vi "objectDB.vi"(7 "Action":T1, 8 "error in (no error)":errorcluster, 9 "timeout in ms (0)":i32, 10 "name":string, 11 "objectRef":refnum<class "HGF_Reference.lvclass">) -> (0 "error out":errorcluster, 1 "obj exists":bool, 2 "name out":string, 3 "objectRef out":refnum<class "HGF_Reference.lvclass">, 4 "object list names":string[](array[string]), 5 "object list refs":refnum<class "HGF_Reference.lvclass">[](array[class]))   [LabVIEW 2012, in "HGF_ObjectManager.lvlib"]
doc: "Functional Global Variable that manages an array of referenced objects by name."
uses:
  HGF_ObjectManager.lvlib
  HGF_BaseClasses/HGF_Reference/HGF_Reference.lvclass
  action.ctl
panel:
  in  "objectType":T2
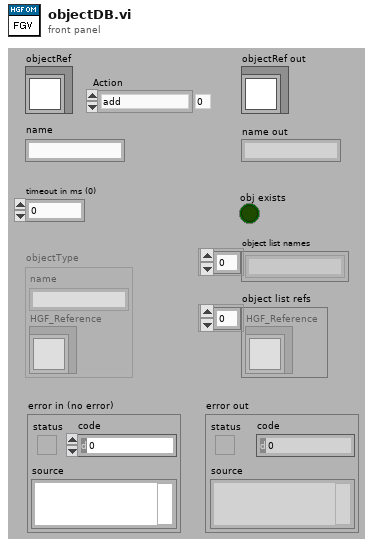
[diagram p1: front panel]
types:
  T1 = typedef "HGF_ObjectManager.lvlib/action.ctl" = enum16{"add", "remove", "name2ref", "ref2name ", "obj exists?", "cleanup", "get object list", "reset"}
  T2 = cluster{"name":string, "HGF_Reference":refnum<class "HGF_Reference.lvclass">}
  T3 = cluster{"name":string, "HGF_Reference":refnum<class "HGF_Reference.lvclass">}[]
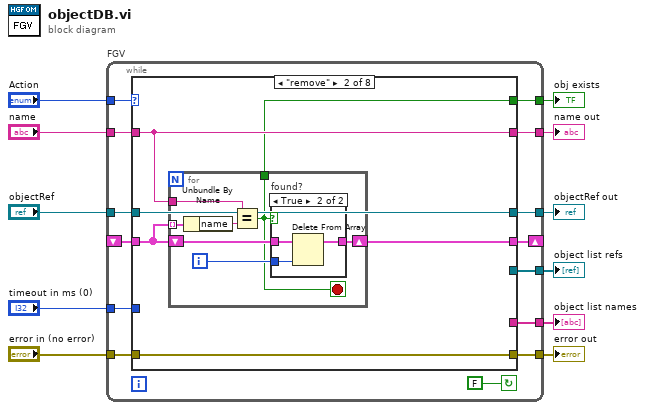
[diagram p0: block diagram]
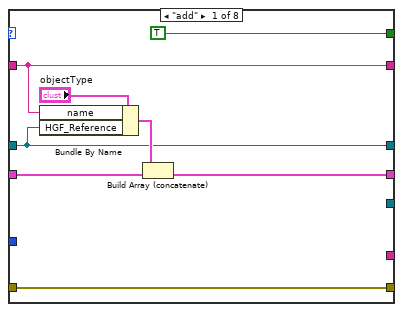
[diagram p2: hidden frame]
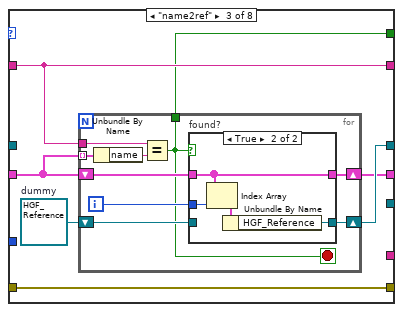
[diagram p4: hidden frame]
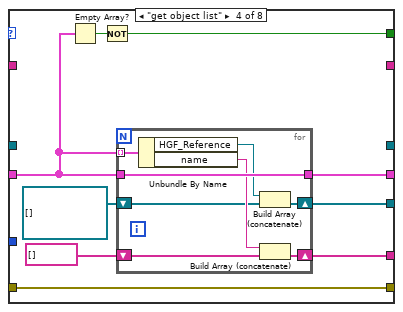
[diagram p6: hidden frame]
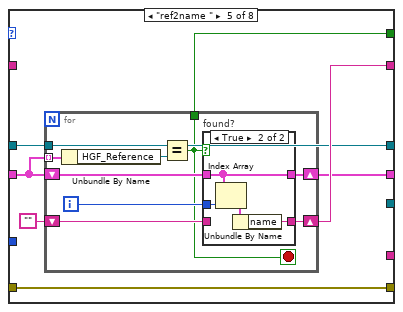
[diagram p7: hidden frame]
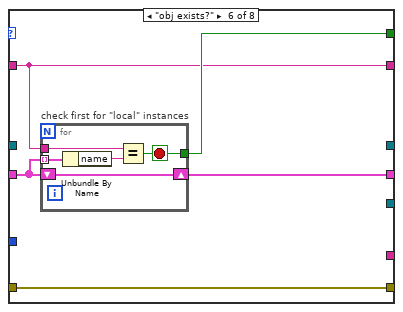
[diagram p9: hidden frame]
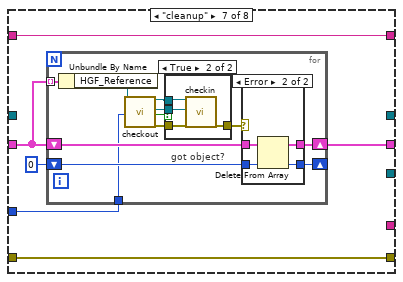
[diagram p10: hidden frame]
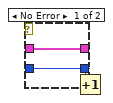
[diagram p12: hidden frame]
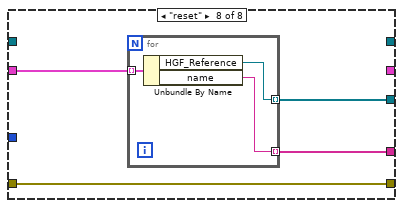
[diagram p13: hidden frame]
diagram:
  n1 = while "FGV" {
    shift-right: [w15] -> _
    shift-left: _ -> [w23]
    tunnel: "name" -> [w25]
    tunnel: "objectRef" -> [w24]
    tunnel: "Action" -> [w22]
    tunnel: [w21] -> w8
    tunnel: [w20] -> w9
    tunnel: [w18] -> w4
    tunnel: [w17] -> w10
    tunnel: [w16] -> w11
    tunnel: "timeout in ms (0)" -> [w14]
    tunnel: "error in (no error)" -> [w13]
    tunnel: [w12] -> w1
    stop <- FALSE continue-if-true
    n2 = case shown="\"remove\"" w22 {
      tunnel: w25 -> [w29 w37 w54 _ _ w113 w124 _]
      tunnel: w24 -> [w30 w36 _ _ w91 _ _ _]
      tunnel: w23 -> [w32 w39 w56 w75 w93 w116 w127 w154]
      tunnel: [w30 w36 w57 _ w91 _ _ _] -> w21
      tunnel: [w29 w37 w54 _ w95 w113 w124 _] -> w20
      tunnel: [TRUE w35 w52 w73 w92 w114 _ _] -> w18
      tunnel: [_ _ _ w79 _ _ _ w152] -> w17
      tunnel: [_ _ _ w78 _ _ _ w153] -> w16
      tunnel: [w31 w38 w55 w81 w94 w115 w126 _] -> w15
      tunnel: w14 -> [_ _ _ _ _ _ w123 _]
      tunnel: w13 -> [w26 w34 w51 w76 w90 w112 w122 w151]
      tunnel: [w26 w34 w51 w76 w90 w112 w122 w151] -> w12
      frame "add" {
        n3 = Bundle By Name(cluster="objectType", "name"=w29, "HGF_Reference"=w30) -> (w33:T2)
        n4 = Build Array (concatenate)(w33, w32) -> (w31:T3)
      }
      frame "remove" {
        n5 = for {
          tunnel: w39 -> [w46] mode=indexing
          tunnel: w37 -> [w45]
          shift-right: [w41] -> w38
          shift-left: w39 -> [w42]
          tunnel: [w40] -> w35
          i -> [w43]
          stop <- w40 stop-if-true
          n6 = Unbundle By Name(w46) -> ("name"=w44:string)
          n7 = Equal?(x=w45, y=w44) -> (x = y?=w40:bool)
          n8 = case "found?" shown="True" w40 {
            tunnel: w42 -> [w47 w50]
            tunnel: w43 -> [_ w48]
            tunnel: [w47 w49] -> w41
            frame False {
            }
            frame True {
              n9 = Delete From Array(array=w50, index=w48) -> (array with subset deleted=w49:T3)  [unwired: 1 in, 1 out]
            }
          }
        }
      }
      frame "name2ref" {
        w53 = refnum<class "HGF_Reference.lvclass"> refnum  # dummy
        n10 = for {
          tunnel: w56 -> [w66] mode=indexing
          tunnel: w54 -> [w65]
          shift-right: [w62] -> w57
          shift-left: w53 -> [w61]
          shift-right: [w60] -> w55
          shift-left: w56 -> [w59]
          tunnel: [w58] -> w52
          i -> [w63]
          stop <- w58 stop-if-true
          n11 = Unbundle By Name(w66) -> ("name"=w64:string)
          n12 = Equal?(x=w65, y=w64) -> (x = y?=w58:bool)
          n13 = case "found?" shown="True" w58 {
            tunnel: w59 -> [w68 w71]
            tunnel: w63 -> [_ w72]
            tunnel: [w68 w71] -> w60
            tunnel: [w67 w70] -> w62
            tunnel: w61 -> [w67 _]
            frame False {
            }
            frame True {
              n14 = Index Array(array=w71, index=w72) -> (element=w69:T2)
              n15 = Unbundle By Name(w69) -> ("HGF_Reference"=w70:refnum<class "HGF_Reference.lvclass">)
            }
          }
        }
      }
      frame "get object list" {
        n16 = Empty Array?(array=w75) -> (empty?=w74:bool)
        n17 = Not(x=w74) -> (.not. x?=w73:bool)
        n18 = for {
          tunnel: w75 -> [w89] mode=indexing
          tunnel: w75 -> [w88]
          tunnel: [w88] -> w81
          shift-right: [w87] -> w79
          shift-left: string[] [] -> [w86]
          shift-right: [w83] -> w78
          shift-left: refnum<class "HGF_Reference.lvclass">[] [] -> [w82]
          n19 = Unbundle By Name(w89) -> ("HGF_Reference"=w84:refnum<class "HGF_Reference.lvclass">, "name"=w85:string)
          n20 = Build Array (concatenate)(w84, w82) -> (w83:refnum<class "HGF_Reference.lvclass">[])
          n21 = Build Array (concatenate)(w85, w86) -> (w87:string[])
        }
      }
      frame "ref2name " {
        n22 = for {
          tunnel: w93 -> [w105] mode=indexing
          shift-right: [w102] -> w95
          shift-left: "" -> [w101]
          tunnel: w91 -> [w100]
          shift-right: [w99] -> w94
          shift-left: w93 -> [w98]
          tunnel: [w97] -> w92
          i -> [w103]
          stop <- w97 stop-if-true
          n23 = Unbundle By Name(w105) -> ("HGF_Reference"=w104:refnum<class "HGF_Reference.lvclass">)
          n24 = Equal?(x=w100, y=w104) -> (x = y?=w97:bool)
          n25 = case "found?" shown="True" w97 {
            tunnel: w98 -> [w107 w110]
            tunnel: w103 -> [_ w111]
            tunnel: [w107 w110] -> w99
            tunnel: [w106 w109] -> w102
            tunnel: w101 -> [w106 _]
            frame False {
            }
            frame True {
              n26 = Index Array(array=w110, index=w111) -> (element=w108:T2)
              n27 = Unbundle By Name(w108) -> ("name"=w109:string)
            }
          }
        }
      }
      frame "obj exists?" {
        n28 = for "check first for \"local\" instances" {
          tunnel: w116 -> [w121] mode=indexing
          tunnel: w113 -> [w119]
          shift-right: [w118] -> w115
          shift-left: w116 -> [w118]
          tunnel: [w117] -> w114
          stop <- w117 stop-if-true
          n29 = Unbundle By Name(w121) -> ("name"=w120:string)
          n30 = Equal?(x=w119, y=w120) -> (x = y?=w117:bool)
        }
      }
      frame "cleanup" {
        n31 = for {
          tunnel: w127 -> [w139] mode=indexing
          shift-right: [w135] -> w126
          shift-left: w127 -> [w138]
          shift-right: [w137] -> _
          shift-left: 0 -> [w136]
          tunnel: w123 -> [w128]
          n32 = Unbundle By Name(w139) -> ("HGF_Reference"=w129:refnum<class "HGF_Reference.lvclass">)
          n33 = call "checkout.vi"("HGF_Reference"=w129, "timeout in ms (-1)"=w128) -> ("dup HGF_Reference"=w134:refnum<class "HGF_Reference.lvclass">, "Object"=w131:refnum<class>, "got object?"=w130:bool, "error out"=w133:errorcluster)  [unwired: 2 in, 12 out]
          n34 = case "got object?" shown="True" w130 {
            tunnel: w134 -> [_ w141]
            tunnel: w133 -> [w140 w144]
            tunnel: [w140 w143] -> w132
            tunnel: w131 -> [_ w142]
            frame False {
            }
            frame True {
              n35 = call "checkin.vi"("HGF_Reference"=w141, "Object"=w142, "error in (no error)"=w144) -> ("error out"=w143:errorcluster)  [unwired: 2 in, 14 out]
            }
          }
          n36 = case shown="Error" w132 {
            tunnel: w138 -> [w147 w150]
            tunnel: [w147 w149] -> w135
            tunnel: w136 -> [w146 w148]
            tunnel: [w145 w148] -> w137
            frame No Error {
              n37 = Increment(x=w146) -> (x+1=w145:i32)
            }
            frame Error {
              n38 = Delete From Array(array=w150, index=w148) -> (array with subset deleted=w149:T3)  [unwired: 1 in, 1 out]
            }
          }
        }
      }
      frame "reset" {
        n39 = for {
          tunnel: w154 -> [w157] mode=indexing
          tunnel: [w156] -> w153 mode=indexing
          tunnel: [w155] -> w152 mode=indexing
          n40 = Unbundle By Name(w157) -> ("HGF_Reference"=w156:refnum<class "HGF_Reference.lvclass">, "name"=w155:string)
        }
      }
    }
  }
  "objectRef out" <- w8
  "name out" <- w9
  "obj exists" <- w4
  "object list names" <- w10
  "object list refs" <- w11
  "error out" <- w1
